vi "Sudoku Calculation Step.vi"(8 "error in (no error)":errorcluster, 11 "Sudoku Class in":refnum<class "Sudoku Class.lvclass">) -> (0 "error out":errorcluster, 2 "Is Modify":bool, 3 "Sudoku Class out":refnum<class "Sudoku Class.lvclass">)   [LabVIEW 2015, in "Sudoku Library.lvlib" / "Sudoku Class.lvclass"]
doc: "Created IvanLis by LabVIEW Portal\nProfile: http://labviewportal.org/memberlist.php?mode=viewprofile&u=987\neMail: IvanLisanov@gMail.com\nTelegram: https://t.me/IvanLis"
uses:
  Sudoku Class.lvclass
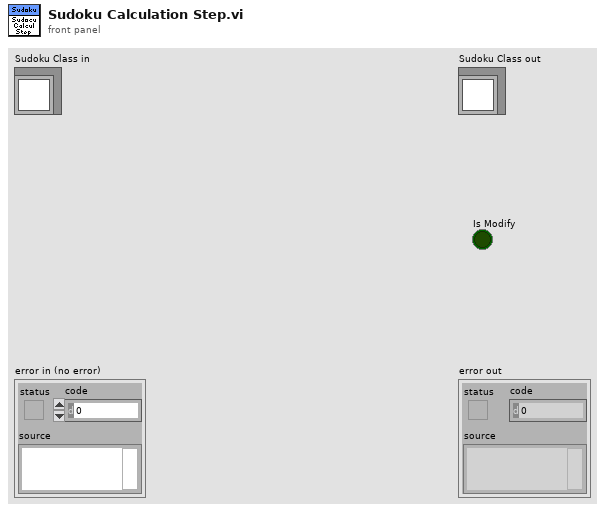
[diagram p1: front panel]
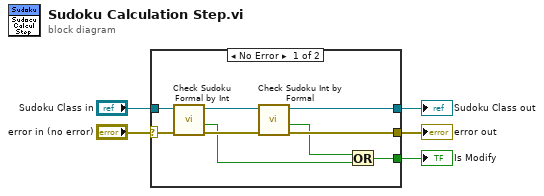
[diagram p0: block diagram]
diagram:
  n1 = case shown="No Error" "error in (no error)" {
    selector: "error in (no error)" -> [w13 w16]
    tunnel: [w11 w16] -> w4
    tunnel: [w12 w15] -> w2
    tunnel: "Sudoku Class in" -> [w14 w15]
    tunnel: [w6 _] -> w1
    frame No Error {
      n2 = call "Check Sudoku Formal by Int.vi"("error in (no error)"=w13, "Sudoku Class in"=w14) -> ("error out"=w9:errorcluster, "Is Modify"=w7:bool, "Sudoku Class out"=w10:refnum<class "Sudoku Class.lvclass">)  [unwired: 6 in, 1 out]
      n3 = call "Check Sudoku Int by Formal.vi"("error in (no error)"=w9, "Sudoku Class in"=w10) -> ("error out"=w11:errorcluster, "Is Modify"=w8:bool, "Sudoku Class out"=w12:refnum<class "Sudoku Class.lvclass">)  [unwired: 6 in, 1 out]
      n4 = Or(x=w8, y=w7) -> (x .or. y?=w6:bool)
    }
    frame Error {
    }
  }
  "error out" <- w4
  "Sudoku Class out" <- w2
  "Is Modify" <- w1
